vi "add_element.vi"   [LabVIEW 2016]
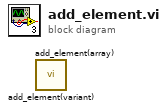
[diagram p0: block diagram]
diagram:
  n1 = call "add_element(variant).vi"() -> ()  [unwired: 10 in, 2 out]
  n2 = call "add_element(array).vi"() -> ()  [unwired: 10 in, 2 out]
